vi "Write Node Controller.vi"(8 "error in (no error)":errorcluster, 10 "Node Controller":refnum<class "Node Controller.lvclass">, 11 "Superior Actor in":refnum<class "Root Actor.lvclass">) -> (0 "error out":errorcluster, 3 "Superior Actor out":refnum<class "Root Actor.lvclass">)   [LabVIEW 2024, in "Root Actor.lvclass"]
uses:
  Root Actor.lvclass
  Actor Assistant/Root Actor Node Controller/Node Controller.lvclass
  Root Actor.lvclass/Root Actor.ctl
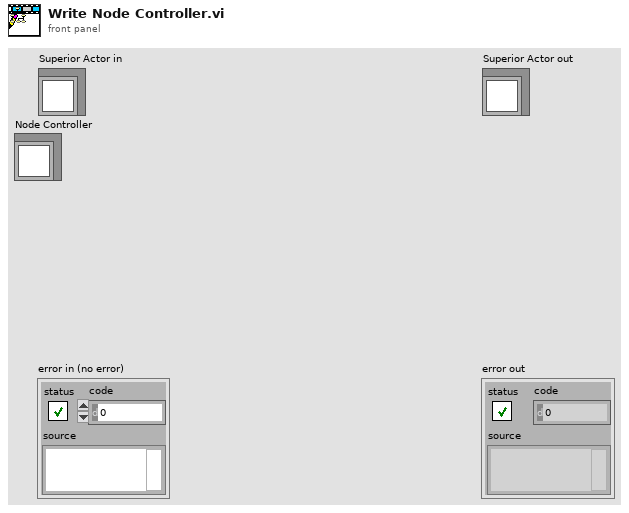
[diagram p1: front panel]
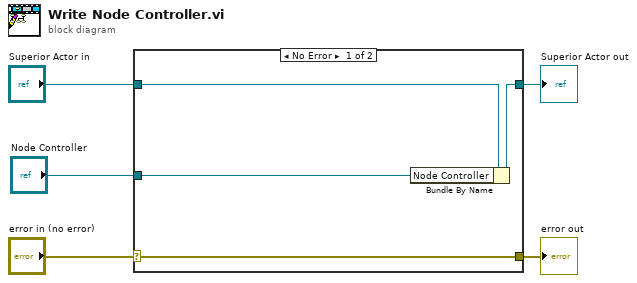
[diagram p0: block diagram]
diagram:
  n1 = case shown="No Error" "error in (no error)" {
    selector: "error in (no error)" -> [w9 w10]
    tunnel: [w9 w10] -> w4
    tunnel: [w7 w11] -> w2
    tunnel: "Superior Actor in" -> [w8 w11]
    tunnel: "Node Controller" -> [w6 _]
    frame No Error {
      n2 = Bundle By Name(cluster=w8, "Node Controller"=w6) -> (w7:refnum<class "Root Actor.lvclass">)
    }
    frame Error {
    }
  }
  "error out" <- w4
  "Superior Actor out" <- w2
